vi "Maxi Gauge-Convert Error2.vi"(3 "Errorwort1":u16) -> (0 "Error Text":string[](array[string]))   [LabVIEW 2013, in "Maxi Gauge.lvlib"]
uses:
  <instrlib>/Maxi Gauge/Maxi Gauge.lvlib
panel:
  in  "Error Tabel":string[][](table)=[["0", "SM1  Measuring Error"], ["1", "SM2  Measuring Error"], ["2", "SM3  Measuring Error"], ["3", "SM4  Measuring Error"], ["4", "SM5  Measuring Error"], ["5", "SM6  Measuring Error"], ["6", ""], ["7", ""], ["8", "SE1 Identify Error"], ["9", "SE2 Identify Error"], ["10", "SE3 Identify Error"], ["11", "SE4 Identify Error"], ["12", "SE5 Identify Error"], ["13", "SE6 Identify Error"], ["14", ""], ["15", ""]]
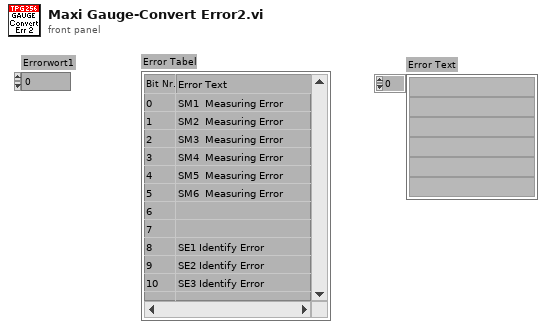
[diagram p1: front panel]
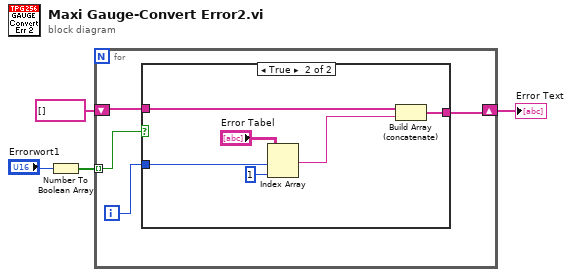
[diagram p0: block diagram]
diagram:
  n1 = Number To Boolean Array(number="Errorwort1") -> (Boolean array=w3:bool[])
  n2 = for {
    tunnel: w3 -> [w8] mode=indexing
    shift-right: [w5] -> w1
    shift-left: string[] [] -> [w6]
    i -> [w7]
    n3 = case shown="True" w8 {
      tunnel: w7 -> [_ w10]
      tunnel: w6 -> [w9 w13]
      tunnel: [w9 w11] -> w5
      frame False {
      }
      frame True {
        n4 = Index Array(array="Error Tabel", index (row)=w10, index (col)=1) -> (element=w12:string)
        n5 = Build Array (concatenate)(w13, w12) -> (w11:string[])
      }
    }
  }
  "Error Text" <- w1
